vi "FGV Logdatei erstellen.vi"(6 "Aktion":T2, 7 "max. Größe  in Byte":i64=31457280, 8 "Pfad Log Datei":path, 9 "Name LogDatei":string, 10 "Logdatei erstellen":T1 items=["Deaktiviert", "Aktiviert"], 11 "Loggen stoppen":bool) -> (0 "Pfad LogDatei neu":path, 1 "Name Log Datei neu":string, 2 "Logdatei erstellen neu":T1 items=["Deaktiviert", "Aktiviert"], 3 "Loggen stoppen":bool, 5 "max. Größe  in Byte neu":i64)   [LabVIEW 2020, in "LogKonfig.lvlib"]
uses:
  LogKonfig.lvlib
  Aktionen Logdatei erstellen.ctl
  Auswahlfeld aktiviert-deaktiviert.ctl
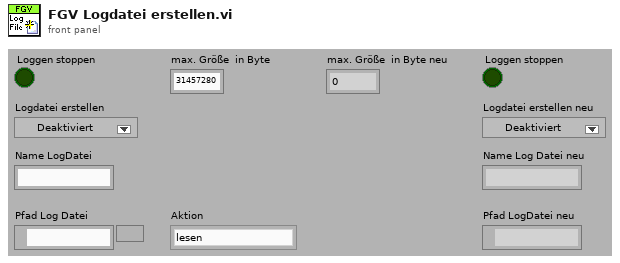
[diagram p1: front panel]
types:
  T1 = typedef "LogKonfig.lvlib/Auswahlfeld aktiviert-deaktiviert.ctl" = u16
  T2 = typedef "LogKonfig.lvlib/Aktionen Logdatei erstellen.ctl" = enum16{"lesen", "Logdatei erstellen NEU", "Name NEU", "Pfad NEU", "Log Stop", "max Size"}
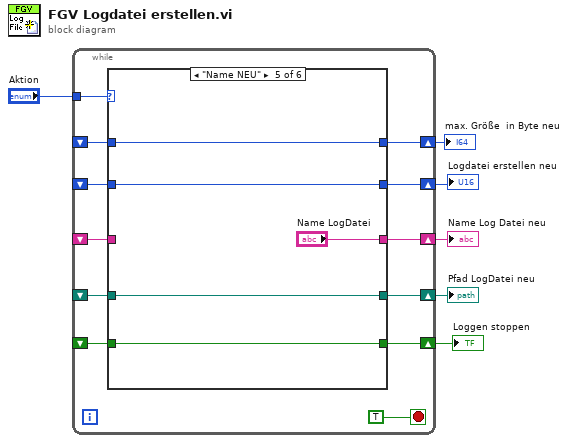
[diagram p0: block diagram]
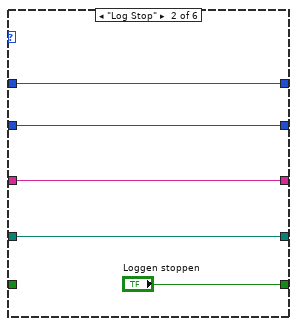
[diagram p3: hidden frame]
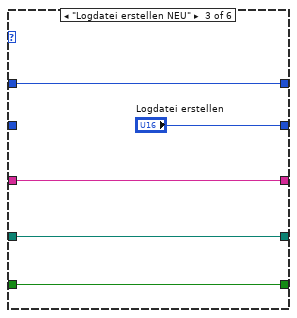
[diagram p4: hidden frame]
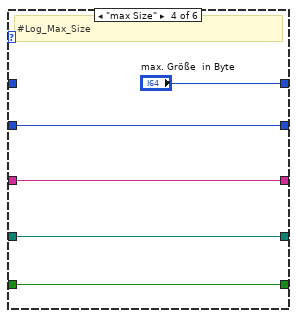
[diagram p5: hidden frame]
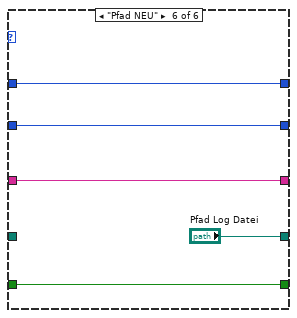
[diagram p6: hidden frame]
diagram:
  n1 = while {
    tunnel: "Aktion" -> [w18]
    shift-right: [w17] -> w3
    shift-left: _ -> [w14]
    shift-right: [w16] -> w5
    shift-left: _ -> [w13]
    shift-right: [w15] -> w4
    shift-left: _ -> [w12]
    shift-right: [w10] -> w2
    shift-left: _ -> [w9]
    shift-right: [w8] -> w1
    shift-left: _ -> [w7]
    stop <- TRUE stop-if-true
    n2 = case shown="\"Name NEU\"" w18 {
      tunnel: [w23 w28 "Logdatei erstellen" w35 w42 w47] -> w17
      tunnel: [w22 w27 w33 w38 "Name LogDatei" w46] -> w16
      tunnel: [w21 w26 w32 w37 w41 "Pfad Log Datei"] -> w15
      tunnel: w14 -> [w23 w28 _ w35 w42 w47]
      tunnel: w13 -> [w22 w27 w33 w38 _ w46]
      tunnel: w12 -> [w21 w26 w32 w37 w41 _]
      tunnel: [w20 "Loggen stoppen" w30 w36 w40 w45] -> w10
      tunnel: w9 -> [w20 _ w30 w36 w40 w45]
      tunnel: [w19 w24 w29 "max. Größe  in Byte" w39 w44] -> w8
      tunnel: w7 -> [w19 w24 w29 _ w39 w44]
      frame "lesen", Default {
      }
      frame "Log Stop" {
      }
      frame "Logdatei erstellen NEU" {
      }
      frame "max Size" {
        # "#Log_Max_Size"
      }
      frame "Name NEU" {
      }
      frame "Pfad NEU" {
      }
    }
  }
  "Name Log Datei neu" <- w5
  "Pfad LogDatei neu" <- w4
  "Logdatei erstellen neu" <- w3
  "Loggen stoppen" <- w2
  "max. Größe  in Byte neu" <- w1
